vi "DB Float Array.vi"() -> (3 "DB Int Array":sgl[](array[numeric]))   [LabVIEW 2023, in "Database.lvlib"]
uses:
  Database.lvlib
  bin/Database.dll
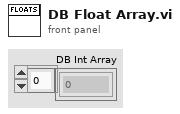
[diagram p1: front panel]
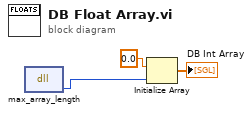
[diagram p0: block diagram]
diagram:
  n1 = dll-call lib="C:/Users/cfangmeier3/Desktop/nebraska-silicon-lab/pixel-gantry-control/Gantry/Shared Components/bin/Database.dll" fn="max_array_length"() -> ("return type"=w2:i32)  [unwired: 3 in, 2 out]
  n2 = Initialize Array(sgl 0.0 ("element"), w2) -> (→"DB Int Array":sgl[])
